vi "New Climb Logic.vi"(8 "Arm Current":dbl, 9 "In Range?":bool, 10 "Limits":cluster{"Base":bool, "Top":bool, "Dummy":bool}, 11 "Climb":bool) -> (0 "Reset Encoder":bool, 1 "Solenoid Value":T1, 2 "Arm Motor":dbl, 3 "Climb State":T2(ring), 4 "Lock":bool, 5 "Arm Set":dbl)   [LabVIEW 2012]
uses:
  <vilib>/Rock Robotics/WPI/Solenoid/WPI_SolenoidValue.ctl
panel:
  out "Numeric":dbl
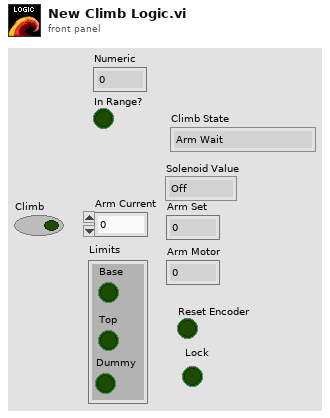
[diagram p1: front panel]
types:
  T1 = typedef "WPI_SolenoidValue.ctl" = enum16{"Off", "On", "Forward", "Reverse"}
  T2 = enum16{"Arm Wait", "Arm Up", "Arm Down", "Arm Attach"}
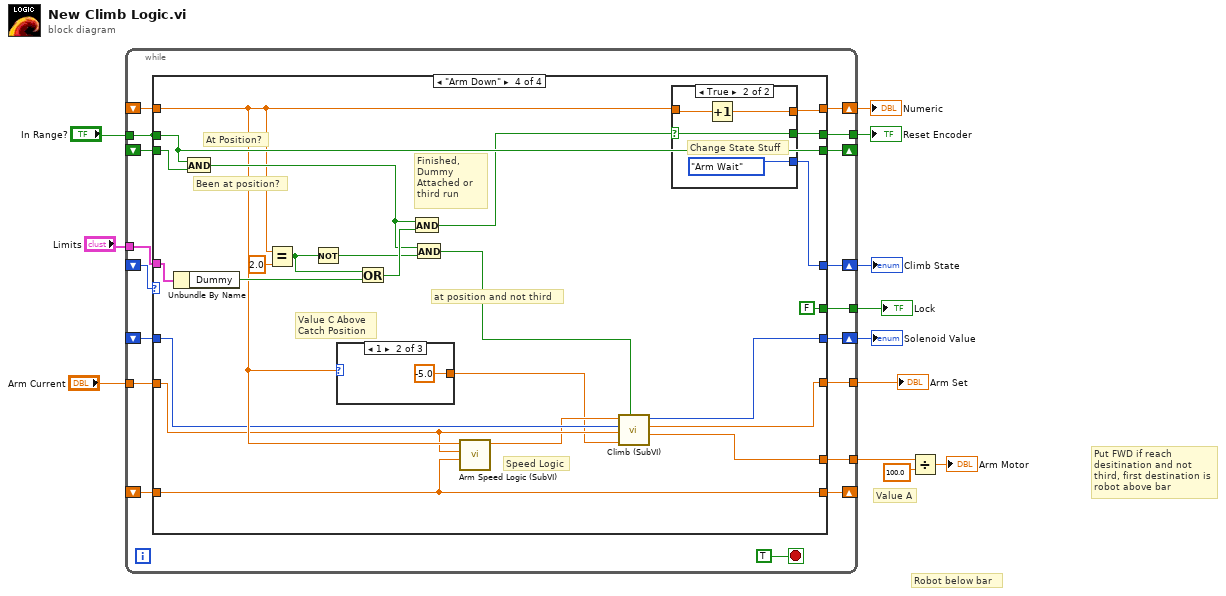
[diagram p0: block diagram]
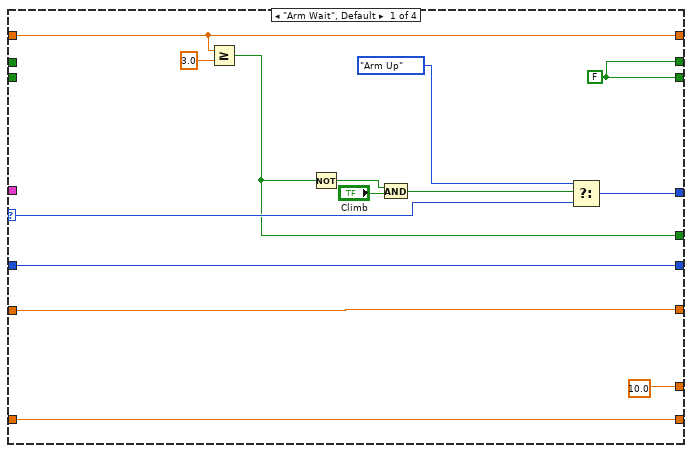
[diagram p2: hidden frame]
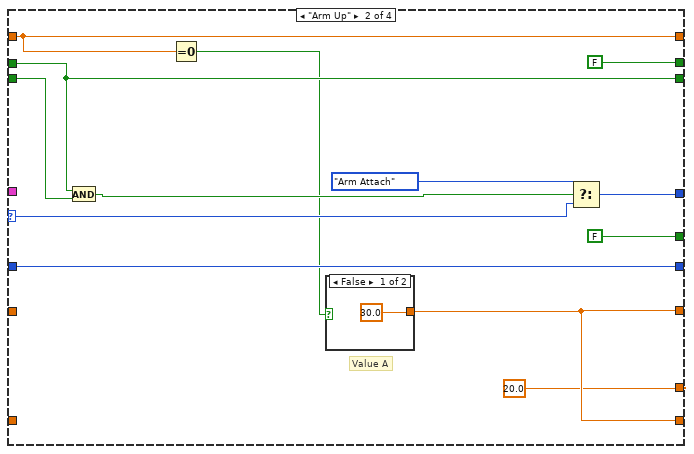
[diagram p3: hidden frame]
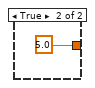
[diagram p4: hidden frame]
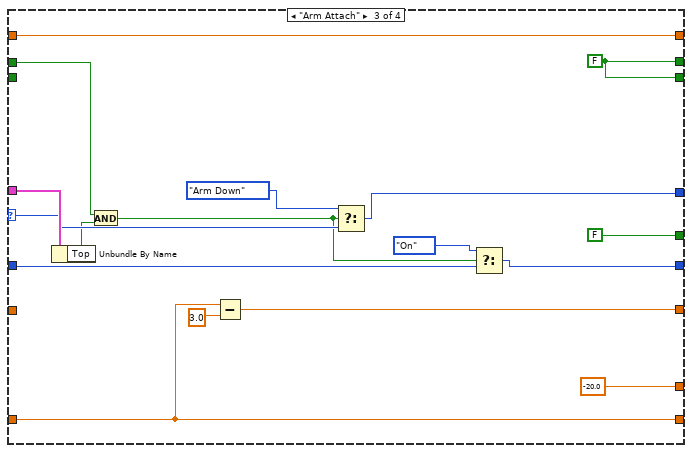
[diagram p5: hidden frame]
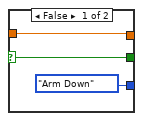
[diagram p6: hidden frame]
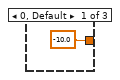
[diagram p7: hidden frame]
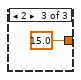
[diagram p8: hidden frame]
diagram:
  # "Put FWD if reach desitination and not third, first destination is robot above bar"
  # "Robot below bar"
  # "Value A"
  n1 = while {
    shift-right: [w30] -> w8
    shift-left: _ -> [w27]
    tunnel: "In Range?" -> [w14]
    shift-right: [w26] -> _
    shift-left: _ -> [w25]
    tunnel: "Limits" -> [w24]
    shift-right: [w23] -> w9
    shift-left: _ -> [w22]
    tunnel: "Arm Current" -> [w21]
    tunnel: [w28] -> w2
    shift-right: [w20] -> w4
    shift-left: _ -> [w19]
    tunnel: [w18] -> w11
    tunnel: [w17] -> w12
    shift-right: [w16] -> _
    shift-left: _ -> [w15]
    tunnel: [w14] -> _
    tunnel: [w13] -> w5
    stop <- TRUE stop-if-true
    n2 = case shown="\"Arm Down\"" w27 {
      selector: w27 -> [w43 w56 w75 _]
      tunnel: [w44 w57 w73 w83] -> w30
      tunnel: [w41 w46 w70 w81] -> w28
      tunnel: w14 -> [_ w53 w68 w91]
      tunnel: [w40 w53 w66 w91] -> w26
      tunnel: w25 -> [_ w51 _ w90]
      tunnel: w24 -> [_ _ w76 w100]
      tunnel: [w31 w52 w63 w99] -> w23
      tunnel: w22 -> [w31 w52 w62 w80]
      tunnel: w21 -> [w41 _ _ w82]
      tunnel: [w39 w50 w65 w86] -> w20
      tunnel: w19 -> [w39 w50 w65 w85]
      tunnel: [w40 FALSE ("At Position") w66 w84] -> w18
      tunnel: [w32 FALSE FALSE FALSE] -> w17
      tunnel: [w34 w46 w71 w97] -> w16
      tunnel: w15 -> [w34 _ w71 w97]
      tunnel: [10.0 ("x") 20.0 ("x") -20.0 ("x") w96] -> w13
      frame "Arm Wait", Default {
        w40 = FALSE ("At Position")
        n3 = Greater Or Equal?(x=w39, y=3.0) -> (x >= y?=w32:bool)
        n4 = Not(x=w32) -> (.not. x?=w35:bool)
        n5 = And(x=w35, y="Climb") -> (x .and. y?=w36:bool)
        n6 = Select(t=T2."Arm Up", s=w36, f=w43) -> (s? t:f=w44:T2)
      }
      frame "Arm Up" {
        # "Value A"
        n7 = And(x=w53, y=w51) -> (x .and. y?=w54:bool)
        n8 = Equal To 0?(x=w50) -> (x = 0?=w47:bool)
        n9 = case shown="False" w47 {
          tunnel: [30.0 ("y") 5.0 ("y")] -> w46
          frame False {
          }
          frame True {
          }
        }
        n10 = Select(t=T2."Arm Attach", s=w54, f=w56) -> (s? t:f=w57:T2)
      }
      frame "Arm Attach" {
        w66 = FALSE
        n11 = Unbundle By Name(w76) -> ("Top"=w67:bool)
        n12 = And(x=w68, y=w67) -> (x .and. y?=w61:bool)
        n13 = Subtract(x=w71, y=3.0) -> (x-y=w70:dbl)
        n14 = Select(t=T2."Arm Down", s=w61, f=w75) -> (s? t:f=w73:T2)
        n15 = Select(t=WPI_SolenoidValue."On" ("y"), s=w61, f=w62) -> (s? t:f=w63:T1)
      }
      frame "Arm Down" {
        # "Speed Logic"
        # "Value C Above Catch Position"
        # "Been at position?"
        # "At Position?"
        # "at position and not third"
        # "Finished, Dummy Attached or third run"
        n16 = Unbundle By Name(w100) -> ("Dummy"=w93:bool)
        n17 = And(x=w91, y=w90) -> (x .and. y?=w89:bool)
        n18 = Equal?(x=w85, y=2.0) -> (x = y?=w92:bool)
        n19 = Not(x=w92) -> (.not. x?=w88:bool)
        n20 = case shown="1" w85 {
          tunnel: [-10.0 ("y") -5.0 ("y") 15.0 ("y")] -> w77
          frame 0, Default {
          }
          frame 1 {
          }
          frame 2 {
          }
        }
        n21 = Or(x=w92, y=w93) -> (x .or. y?=w94:bool)
        n22 = And(x=w89, y=w94) -> (x .and. y?=w87:bool)
        n23 = And(x=w89, y=w88) -> (x .and. y?=w79:bool)
        n24 = call "Arm Speed Logic (SubVI).vi"("y"=w97, "Arm Current"=w82, "Numeric"=w85) -> ("f"=w78:dbl)  [unwired: 8 in]
        n25 = call "Climb (SubVI).vi"("At position and not third"=w79, "C"=w77, "Arm Current"=w82, "Solenoid in"=w80, "Input from Speed logic"=w78) -> ("Arm Motor"=w96:dbl, "Arm Set"=w81:dbl, "Solenoid out"=w99:T1)  [unwired: 4 in]
        n26 = case shown="True" w87 {
          selector: w87 -> [w102 w105]
          tunnel: w85 -> [w103 w106]
          tunnel: [w103 w107] -> w86
          tunnel: [w102 w105] -> w84
          tunnel: [T2."Arm Down" ("t") T2."Arm Wait" ("t")] -> w83
          frame False {
          }
          frame True {
            # "Change State Stuff"
            n27 = Increment(x=w106) -> (x+1=w107:dbl)
          }
        }
      }
    }
  }
  "Arm Set" <- w2
  "Climb State" <- w8
  "Solenoid Value" <- w9
  "Reset Encoder" <- w11
  "Lock" <- w12
  "Numeric" <- w4
  n28 = Divide(x=w5, y=100.0) -> (x/y=→"Arm Motor":dbl)
